vi "Read Exception Status1.vi"(7 "Unit_ID":T1, 8 "error in (no error)":errorcluster, 11 "Modbus master in":refnum<class "TCP.lvclass">) -> (0 "error out":errorcluster, 2 "exception status":u8, 3 "Modbus master out":refnum<class "TCP.lvclass">)   [LabVIEW 2019, in "NI_modbus_upd.lvlib"]
doc: "Reads the exception status of a Modbus slave. The exception status is a set of eight status bits. Each status bit represents an exception."
uses:
  NI_modbus_upd.lvlib
  TCP/TCP.lvclass
  Ctl/Unit_ID.ctl
  TCP/TCP.lvclass/TCP.ctl
  Error Generator1.vi
  Function code mismatch error1.vi
  Read ADU Packet Master.vi
  Write ADU Packet Master.vi
  Modbus Data Unit (PDU)/Construct PDU1.vi
  Modbus Data Unit (PDU)/Unflatten to PDU1.vi
  TCP/Protocol Read.vi
  TCP/Protocol Write.vi
  <vilib>/Utility/error.llb/Error Cluster From Error Code.vi
  Modbus Data Unit (PDU)/Deconstruct PDU1.vi
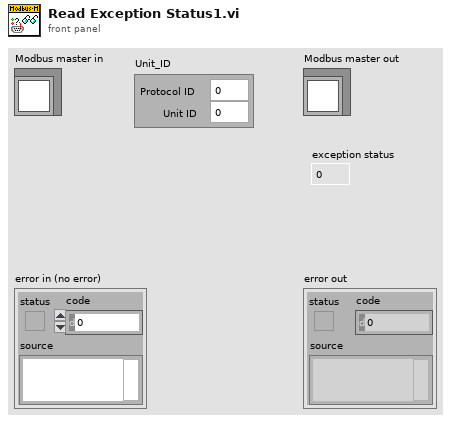
[diagram p1: front panel]
types:
  T1 = typedef "NI_modbus_upd.lvlib/Unit_ID.ctl" = cluster{"Protocol ID":u16, "Unit ID":u8}
  T2 = typedef "NI_modbus_upd.lvlib/MB Modbus Data Unit.ctl" = cluster{"function":T3, "Data":u8[]}
  T3 = typedef "NI_modbus_upd.lvlib/Function.ctl" = u8
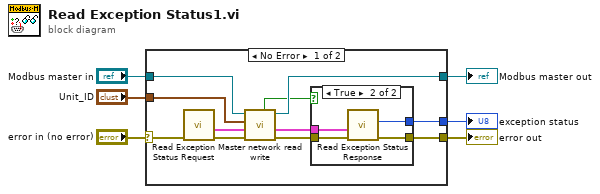
[diagram p0: block diagram]
diagram:
  n1 = case shown="No Error" "error in (no error)" {
    selector: "error in (no error)" -> [w13 w23]
    tunnel: [w17 w24] -> w6
    tunnel: "Modbus master in" -> [w14 w24]
    tunnel: [w16 _] -> w4
    tunnel: [w15 w23] -> w3
    tunnel: "Unit_ID" -> [w7 _]
    frame No Error {
      n2 = call "Read Exception Status Request.vi"("error in (no error)"=w13) -> ("error out"=w12:errorcluster, "Modbus Data Unit out"=w9:T2)  [unwired: 9 in]
      n3 = call "Master network read write.vi"("error in (no error)"=w12, "Modbus Data Unit"=w9, "Unit_ID"=w7, "TCP in"=w14) -> ("error out"=w11:errorcluster, "Modbus data unit out"=w8:T2, "TCP out"=w17:refnum<class "TCP.lvclass">, "PDU valid?"=w10:bool)  [unwired: 4 in]
      n4 = case shown="True" w10 {
        tunnel: [_ w22] -> w16
        tunnel: w11 -> [w18 w21]
        tunnel: [w18 w20] -> w15
        tunnel: w8 -> [_ w19]
        frame False {
        }
        frame True {
          n5 = call "Read Exception Status Response.vi"("error in (no error)"=w21, "Modbus Data Unit in"=w19) -> ("error out"=w20:errorcluster, "exception status"=w22:u8)  [unwired: 8 in]
        }
      }
    }
    frame Error {
    }
  }
  "error out" <- w3
  "Modbus master out" <- w6
  "exception status" <- w4
